vi "Store Static VI References for Subpanel.vi"(8 "error in (no error)":errorcluster, 11 "Example Configuration Dialog in":refnum<class "Example Configuration Dialog.lvclass">) -> (0 "error out":errorcluster, 3 "Example Configuration Dialog out":refnum<class "Example Configuration Dialog.lvclass">)   [LabVIEW 2017, in "Example Configuration Dialog.lvlib" / "Example Configuration Dialog.lvclass"]
uses:
  Example Configuration Dialog.lvclass
  \\Mac\Home/Documents/Extensible-Config-Dialog/Configuration.lvclass
  Configuration.lvclass
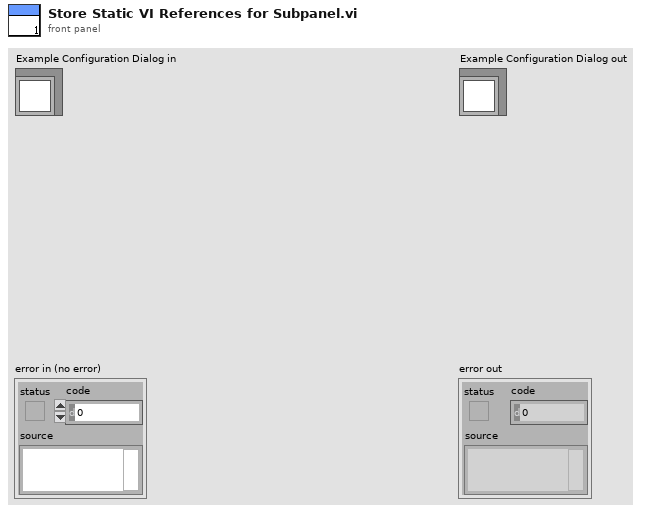
[diagram p1: front panel]
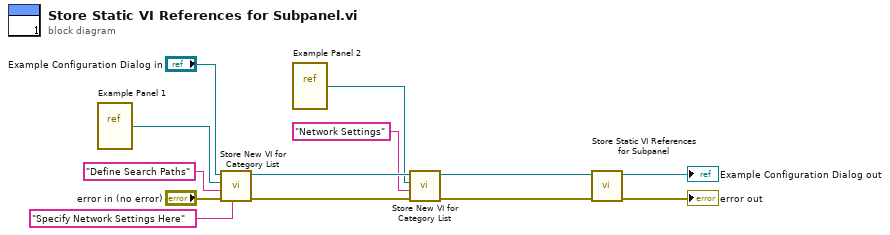
[diagram p0: block diagram]
diagram:
  n1 = vi-ref "Example Panel 1.vi"() -> (w7:refnum<vi>)
  n2 = call "Store New VI for Category List.vi"("Help Text"="Specify Network Settings Here", "error in (no error)"="error in (no error)", "String"="Define Search Paths", "VI Refnum"=w7, "Configuration in"="Example Configuration Dialog in") -> ("error out"=w3:errorcluster, "Configuration out"=w10:refnum<class "Example Configuration Dialog.lvclass">)  [unwired: 5 in]
  n3 = vi-ref "Example Panel 2.vi"() -> (w8:refnum<vi>)
  n4 = call "Store New VI for Category List.vi"("error in (no error)"=w3, "String"="Network Settings", "VI Refnum"=w8, "Configuration in"=w10) -> ("error out"=w4:errorcluster, "Configuration out"=w9:refnum<class "Example Configuration Dialog.lvclass">)  [unwired: 6 in]
  n5 = call-parent "Store Static VI References for Subpanel.vi"("error in (no error)"=w4, "Configuration in"=w9) -> ("error out"=→"error out":errorcluster, "Configuration out"=→"Example Configuration Dialog out":refnum<class "Example Configuration Dialog.lvclass">)  [unwired: 8 in]
